vi "Tree Config Data From Tree.vi"(7 "Parent Path":path, 8 "error in":errorcluster, 11 "XML in":string) -> (0 "error out":errorcluster, 1 "Test Base Paths":T1[](array[typedef]), 2 "Test Config Data":T2[](array[typedef]) {"Test Ranking" items=["Low", "Normal", "High"]}, 3 "XML out":string)   [LabVIEW 2020]
uses:
  <vilib>/addons/analyzer/_analyzerctrls.llb/VIAnCtl Test Config Data.ctl
  <vilib>/addons/analyzer/_analyzerctrls.llb/VIAnCtl TestRanking.ctl
  <vilib>/addons/analyzer/_analyzerctrls.llb/VIAnCtl Config Control Value.ctl
  <vilib>/addons/analyzer/_vianuishared.llb/VIAnUI Test Base Path.ctl
  <vilib>/addons/analyzer/_vianuishared.llb/VIAnUI CFG File Info Global.vi
  <vilib>/addons/analyzer/XML Parsing/NI_VIAn_XML Parsing.lvlib
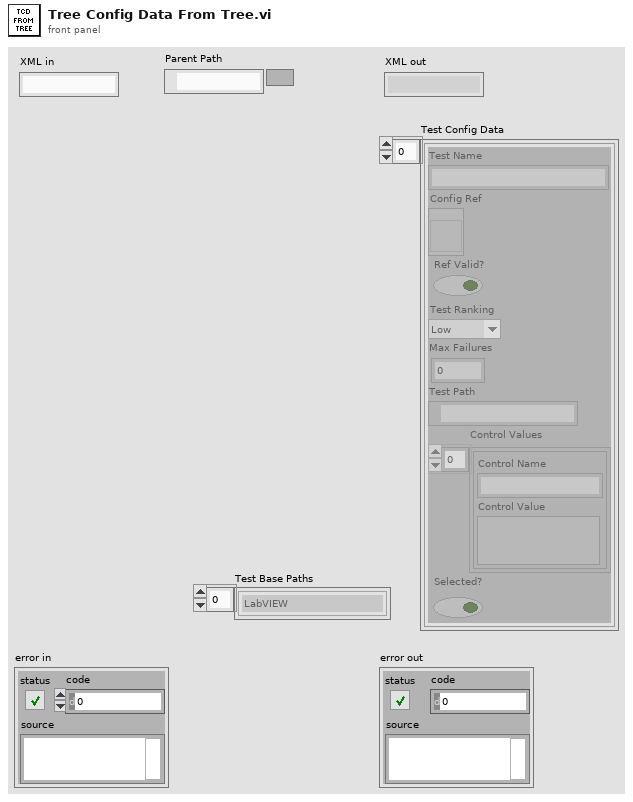
[diagram p1: front panel]
types:
  T1 = typedef "VIAnUI Test Base Path.ctl" = enum16{"LabVIEW", "LabVIEW Data"}
  T2 = typedef "VIAnCtl Test Config Data.ctl" = cluster{"Test Name":string, "Config Ref":refnum<vi>, "Ref Valid?":bool, "Test Ranking":T3, "Max Failures":u32, "Test Path":path, "Control Values":T4[], "Selected?":bool}
  T3 = typedef "VIAnCtl TestRanking.ctl" = u16
  T4 = typedef "VIAnCtl Config Control Value.ctl" = cluster{"Control Name":string, "Control Value":variant}
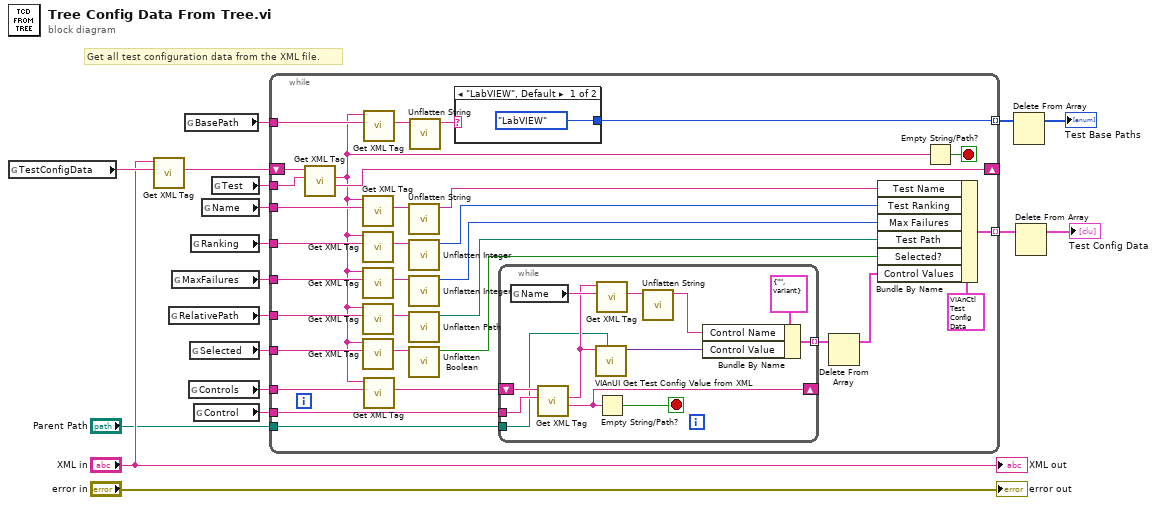
[diagram p0: block diagram]
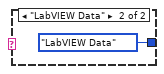
[diagram p2: hidden frame]
diagram:
  # "Get all test configuration data from the XML file."
  n1 = global read "VIAnUI CFG File Info Global.vi" "TestConfigData"() -> (w12:string)
  n2 = call <vilib>:"Get XML Tag.vi"("Tag name"=w12, "XML String in"="XML in") -> ("Tag value"=w17:string)  [unwired: 5 in, 4 out]
  n3 = global read "VIAnUI CFG File Info Global.vi" "RelativePath"() -> (w8:string)
  n4 = global read "VIAnUI CFG File Info Global.vi" "MaxFailures"() -> (w9:string)
  n5 = global read "VIAnUI CFG File Info Global.vi" "BasePath"() -> (w6:string)
  n6 = global read "VIAnUI CFG File Info Global.vi" "Controls"() -> (w3:string)
  n7 = global read "VIAnUI CFG File Info Global.vi" "Selected"() -> (w7:string)
  n8 = global read "VIAnUI CFG File Info Global.vi" "Ranking"() -> (w13:string)
  n9 = global read "VIAnUI CFG File Info Global.vi" "Control"() -> (w2:string)
  n10 = global read "VIAnUI CFG File Info Global.vi" "Name"() -> (w14:string)
  n11 = global read "VIAnUI CFG File Info Global.vi" "Test"() -> (w15:string)
  n12 = while {
    tunnel: [w42] -> w16 mode=indexing
    shift-right: [w49] -> _
    shift-left: w17 -> [w50]
    tunnel: w15 -> [w48]
    tunnel: w14 -> [w46]
    tunnel: w13 -> [w45]
    tunnel: w9 -> [w38]
    tunnel: w8 -> [w35]
    tunnel: w7 -> [w32]
    tunnel: w6 -> [w28]
    tunnel: [w26] -> w5 mode=indexing
    tunnel: w3 -> [w24]
    tunnel: w2 -> [w20]
    tunnel: "Parent Path" -> [w19]
    stop <- w47 stop-if-true
    n13 = call <vilib>:"Get XML Tag.vi"("Tag name"=w48, "XML String in"=w50) -> ("Remaining string"=w49:string, "Tag value"=w25:string)  [unwired: 5 in, 3 out]
    n14 = call <vilib>:"Get XML Tag.vi"("Tag name"=w46, "XML String in"=w25) -> ("Tag value"=w44:string)  [unwired: 5 in, 4 out]
    n15 = call <vilib>:"Get XML Tag.vi"("Tag name"=w45, "XML String in"=w25) -> ("Tag value"=w40:string)  [unwired: 5 in, 4 out]
    n16 = call <vilib>:"Get XML Tag.vi"("Tag name"=w38, "XML String in"=w25) -> ("Tag value"=w37:string)  [unwired: 5 in, 4 out]
    n17 = call <vilib>:"Get XML Tag.vi"("Tag name"=w35, "XML String in"=w25) -> ("Tag value"=w34:string)  [unwired: 5 in, 4 out]
    n18 = call <vilib>:"Get XML Tag.vi"("Tag name"=w32, "XML String in"=w25) -> ("Tag value"=w31:string)  [unwired: 5 in, 4 out]
    n19 = call <vilib>:"Get XML Tag.vi"("Tag name"=w28, "XML String in"=w25) -> ("Tag value"=w29:string)  [unwired: 5 in, 4 out]
    n20 = call <vilib>:"Get XML Tag.vi"("Tag name"=w24, "XML String in"=w25) -> ("Tag value"=w23:string)  [unwired: 5 in, 4 out]
    n21 = call <vilib>:"Unflatten String.vi"("Tag value"=w44) -> ("String"=w41:string)  [unwired: 10 in]
    n22 = call <vilib>:"Unflatten Integer.vi"("Tag value"=w40) -> ("Numeric"=w39:i32)  [unwired: 10 in]
    n23 = call <vilib>:"Unflatten Integer.vi"("Tag value"=w37) -> ("Numeric"=w36:i32)  [unwired: 10 in]
    n24 = call <vilib>:"Unflatten Path.vi"("Tag value"=w34) -> ("Path"=w33:path)  [unwired: 10 in]
    n25 = call <vilib>:"Unflatten Boolean.vi"("Tag value"=w31) -> ("Boolean"=w30:bool)  [unwired: 10 in]
    n26 = call <vilib>:"Unflatten String.vi"("Tag value"=w29) -> ("String"=w27:string)  [unwired: 10 in]
    n27 = case shown="\"LabVIEW\", Default" w27 {
      tunnel: [VIAnUI_Test_Base_Path."LabVIEW" ("Test Base Path") VIAnUI_Test_Base_Path."LabVIEW Data" ("Test Base Path")] -> w26
      frame "LabVIEW", Default {
      }
      frame "LabVIEW Data" {
      }
    }
    n28 = while {
      shift-right: [w58] -> _
      shift-left: w23 -> [w60]
      tunnel: [w61] -> w22 mode=indexing
      tunnel: w20 -> [w59]
      tunnel: w19 -> [w51]
      stop <- w57 stop-if-true
      n29 = global read "VIAnUI CFG File Info Global.vi" "Name"() -> (w56:string)
      n30 = call <vilib>:"Get XML Tag.vi"("Tag name"=w59, "XML String in"=w60) -> ("Remaining string"=w58:string, "Tag value"=w54:string)  [unwired: 5 in, 3 out]
      n31 = call <vilib>:"VIAnUI Get Test Config Value from XML.vi"("Parent Path"=w51, "Control XML"=w54) -> ("Control Value"=w55:variant)  [unwired: 9 in]
      n32 = call <vilib>:"Get XML Tag.vi"("Tag name"=w56, "XML String in"=w54) -> ("Tag value"=w53:string)  [unwired: 5 in, 4 out]
      n33 = Empty String/Path?(string/path=w58) -> (empty?=w57:bool)
      n34 = call <vilib>:"Unflatten String.vi"("Tag value"=w53) -> ("String"=w52:string)  [unwired: 10 in]
      n35 = Bundle By Name(cluster=T4 {"Control Name"="", "Control Value"=variant} ("Config Control Value"), "Control Name"=w52, "Control Value"=w55) -> (w61:T4)
    }
    n36 = Delete From Array(array=w22) -> (array with subset deleted=w21:T4[])  [unwired: 2 in, 1 out]
    n37 = Bundle By Name(cluster=T2 {"Test Name"="", "Config Ref"=refnum, "Ref Valid?"=FALSE, "Test Ranking"=0, "Max Failures"=0, "Test Path"=path "", "Control Values"=[], "Selected?"=FALSE} ("Cluster"), "Test Name"=w41, "Test Ranking"=w39, "Max Failures"=w36, "Test Path"=w33, "Selected?"=w30, "Control Values"=w21) -> (w42:T2)
    n38 = Empty String/Path?(string/path=w25) -> (empty?=w47:bool)
  }
  n39 = Delete From Array(array=w5) -> (array with subset deleted=→"Test Base Paths":T1[])  [unwired: 2 in, 1 out]
  n40 = Delete From Array(array=w16) -> (array with subset deleted=→"Test Config Data":T2[])  [unwired: 2 in, 1 out]
  "error out" <- "error in"
  "XML out" <- "XML in"
